vi "Copy To IMAQ.vi"() -> ()   [LabVIEW 2020]
uses:
  LabVIEW/g_ar_toolkit.image/Raw Memory Information.ctl
  LabVIEW/g_ar_toolkit.image/Raw Memory Information Dimension.ctl
  LabVIEW/g_ar_toolkit.image/DrawImageToPictureARGB.vi
  LabVIEW/g_ar_toolkit.image/NewImageARGB.vi/3321fa97-f432-4e1e-8db9-a0df79aed21b.vi
  LabVIEW/g_ar_toolkit.image/ARGB Colour to U32 Pixel Value.vi
  LabVIEW/g_ar_toolkit.image/DrawImageToPictureARGB.vi/8cd07b1b-062e-4fe4-9e87-2eb3dc89fe0e.vi
  LabVIEW/g_ar_toolkit.image/CopyImageToRawMemoryARGB.vi/01eda17f-9221-4e43-bf47-cf9d986167a3.vi
  LabVIEW/g_ar_toolkit.common/Module Path.vi
  <vilib>/Utility/error.llb/Error Cluster From Error Code.vi
  <vilib>/vision/EDVR.llb/IMAQ ImageToEDVR 2D U32.vi
  LabVIEW/g_ar_toolkit.image/g_ar_toolkit.image.lvlib
  LabVIEW/g_ar_toolkit.image/NewImageARGBArray.vi
panel:
  in  "Mode":T1(ring)
  out "IMAQ":T2(plugin-control)
  out "Input":picture
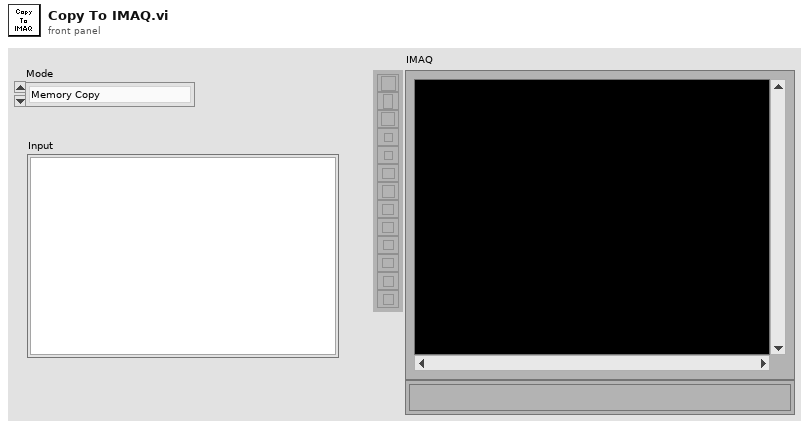
[diagram p1: front panel]
types:
  T1 = enum16{"Memory Copy", "EDVR Access", "Array Values"}
  T2 = typedef "IMAQ Image.ctl" = refnum<image>
  T3 = typedef "Image Type" = u32
  T4 = typedef "g_ar_toolkit.image.lvlib/ARGB Image.ctl" = refnum<data-value>
  T5 = enum32{"Map Pixel Pointer", "Unmap Pixel Pointer", "Get Pixels Infos"}
  T6 = typedef "g_ar_toolkit.image.lvlib/Raw Memory Information.ctl" = cluster{"Memory Address":u64, "Dimension 0":T7, "Dimension 1":T7}
  T7 = typedef "g_ar_toolkit.image.lvlib/Raw Memory Information Dimension.ctl" = cluster{"Size":u16, "Stride":u32}
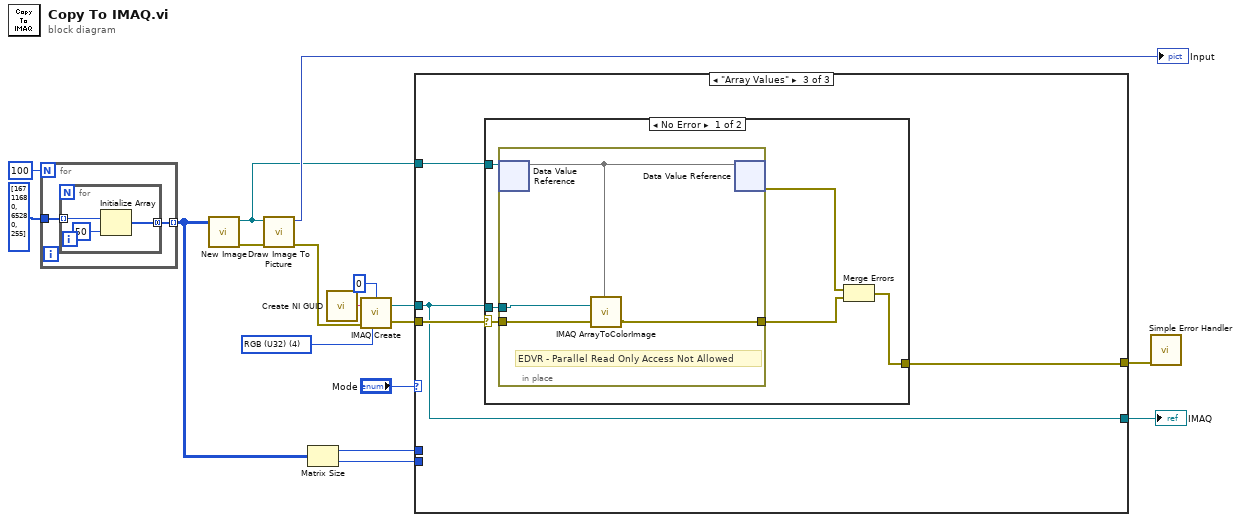
[diagram p0: block diagram]
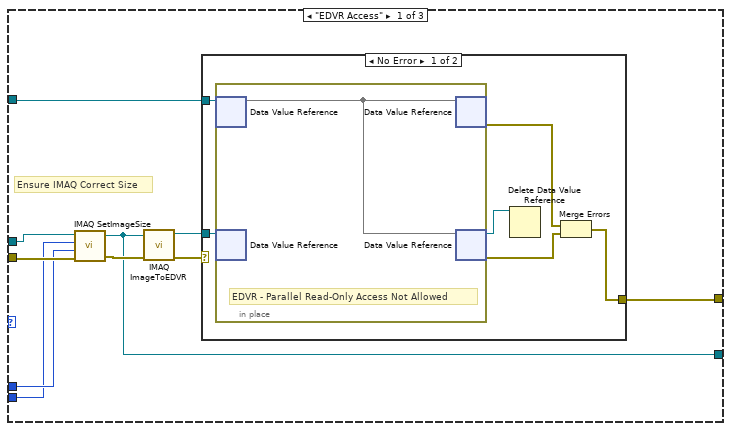
[diagram p2: hidden frame]
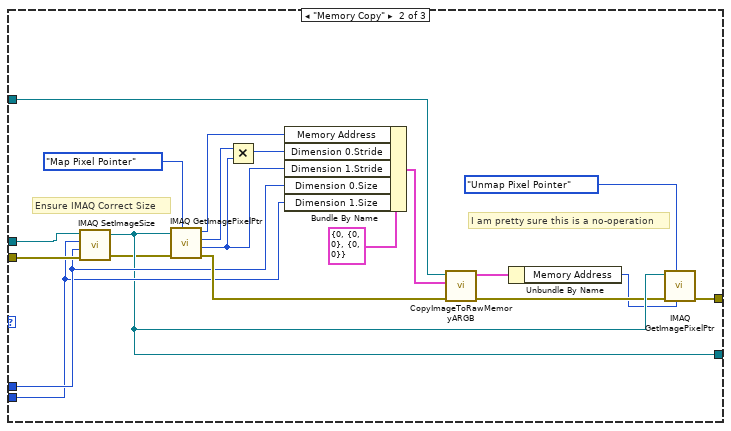
[diagram p4: hidden frame]
diagram:
  w15 = T3 4 items=["Grayscale (U8)", "Grayscale (I16)", "Grayscale (SGL)", "Complex (CSG)", "RGB (U32)", "HSL (U32)", "RGB (U64)", "Grayscale (U16)"] ("Image Type")
  n1 = for {
    N: 100 -> [_]
    tunnel: u32[] [16711680, 65280, 255] ("color(black)") -> [w19]
    tunnel: [w18] -> w1 mode=indexing
    n2 = for {
      tunnel: w19 -> [w22] mode=indexing
      tunnel: [w20] -> w18 mode=concatenating
      n3 = Initialize Array(w22, 50 ("dimension size")) -> (w20:u32[])
    }
  }
  n4 = call-poly "New Image.vi"("U32 ARBG Data  (Default: Empty)"=w1) -> ("error out"=w3:errorcluster, "New ARGB Image"=w2:T4)  [unwired: 9 in]
  n5 = call-poly "Draw Image To Picture.vi"("error in (no error)"=w3, "ARGB Image Source"=w2) -> ("error out"=w9:errorcluster, "Picture"=→"Input":picture)  [unwired: 8 in]
  n6 = Matrix Size(0:w1) -> (1:w11:i32, 2:w10:i32)
  n7 = call <vilib>:"Create NI GUID.vi"() -> ("NI GUID"=w5:string)
  n8 = call "IMAQ Create"("Border Size"=0, "Image Name"=w5, "Image Type"=w15, "error in (no error)"=w9) -> ("New Image"=w12:T2, "error out"=w13:errorcluster)  [unwired: 1 in]
  n9 = case shown="\"Array Values\"" "Mode" {
    tunnel: w13 -> [w29 w59 w64]
    tunnel: w12 -> [w28 w58 w61]
    tunnel: w11 -> [w24 w57 _]
    tunnel: w10 -> [w23 w56 _]
    tunnel: [w26 w55 w61] -> w7
    tunnel: [w27 w54 w62] -> w6
    tunnel: w2 -> [w25 w53 w63]
    frame "EDVR Access" {
      # "Ensure IMAQ Correct Size"
      n10 = call "IMAQ SetImageSize"("error in (no error)"=w29, "Y Resolution"=w24, "X Resolution"=w23, "Image"=w28) -> ("error out"=w32:errorcluster, "Image Out"=w26:T2)  [unwired: 1 in]
      n11 = call-poly <vilib>:"IMAQ ImageToEDVR.vi"("error out"=w32, "Image"=w26) -> ("error out"=w30:errorcluster, "EDVR 2D U32"=w31:refnum<data-value>)  [unwired: 7 in, 1 out]
      n12 = case shown="No Error" w30 {
        selector: w30 -> [_ w40]
        tunnel: w31 -> [w38 _]
        tunnel: [w34 w40] -> w27
        tunnel: w25 -> [w33 _]
        frame No Error {
          n13 = in-place {
            # "EDVR - Parallel Read-Only Access Not Allowed"
            n14 = in-place-dvr #1(w33) -> (w39:u32[][])  [unwired: 1 out]
            n15 = in-place-dvr #2(w38) -> ()  [unwired: 2 out]
            n16 = in-place-dvr #1(w39) -> (w36:errorcluster)  [unwired: 1 out]
            n17 = in-place-dvr #2(w39) -> (w37:refnum<data-value>, w35:errorcluster)
          }
          n18 = Delete Data Value Reference(data value reference=w37) -> ()  [unwired: 1 in, 2 out]
          n19 = Merge Errors(w36, w35) -> (w34:errorcluster)
        }
        frame Error {
        }
      }
    }
    frame "Memory Copy" {
      # "Ensure IMAQ Correct Size"
      # "I am pretty sure this is a no-operation"
      n20 = call "IMAQ SetImageSize"("error in (no error)"=w59, "Y Resolution"=w57, "X Resolution"=w56, "Image"=w58) -> ("error out"=w47:errorcluster, "Image Out"=w55:T2)  [unwired: 1 in]
      n21 = call "IMAQ GetImagePixelPtr"("Function"=T5."Map Pixel Pointer", "error in (no error)"=w47, "Image"=w55) -> ("error out"=w60:errorcluster, "Pixel Size (Bytes)"=w41:i32, "LineWidth(Pixels)"=w49:i32, "Pixel Pointer out"=w52:u64)  [unwired: 3 in, 2 out]
      n22 = Multiply(x=w49, y=w41) -> (x*y=w42:i32)
      n23 = Bundle By Name(cluster=T6 {"Memory Address"=0, "Dimension 0"={"Size"=0, "Stride"=0}, "Dimension 1"={"Size"=0, "Stride"=0}} ("Source"), "Memory Address"=w52, "Dimension 0.Stride"=w42, "Dimension 1.Stride"=w41, "Dimension 0.Size"=w57, "Dimension 1.Size"=w56) -> (w46:T6)
      n24 = call "CopyImageToRawMemoryARGB.vi"("error in (no error)"=w60, "Destination"=w46, "ARGB Image Source"=w53) -> ("error out"=w45:errorcluster, "Destination (Duplcate)"=w44:T6)  [unwired: 7 in]
      n25 = Unbundle By Name(w44) -> ("Memory Address"=w43:u64)
      n26 = call "IMAQ GetImagePixelPtr"("Pixel Pointer in"=w43, "Function"=T5."Unmap Pixel Pointer", "error in (no error)"=w45, "Image"=w55) -> ("error out"=w54:errorcluster)  [unwired: 2 in, 5 out]
    }
    frame "Array Values" {
      n27 = case shown="No Error" w64 {
        selector: w64 -> [w66 w75]
        tunnel: w63 -> [w70 _]
        tunnel: [w68 w75] -> w62
        tunnel: w61 -> [w67 _]
        frame No Error {
          n28 = in-place {
            in-place-border: w67 -> [w74]
            in-place-border: w66 -> [w73]
            in-place-border: [w71] -> w65
            # "EDVR - Parallel Read Only Access Not Allowed"
            n29 = in-place-dvr #3(w70) -> (w72:u32[][])  [unwired: 1 out]
            n30 = call "IMAQ ArrayToColorImage"("Image Pixels (U32)"=w72, "Image"=w74, "error in (no error)"=w73) -> ("error out"=w71:errorcluster)  [unwired: 2 in, 1 out]
            n31 = in-place-dvr #3(w72) -> (w69:errorcluster)  [unwired: 1 out]
          }
          n32 = Merge Errors(w69, w65) -> (w68:errorcluster)
        }
        frame Error {
        }
      }
    }
  }
  "IMAQ" <- w7
  n33 = call <vilib>:"Simple Error Handler.vi"("error in (no error)"=w6) -> ()  [unwired: 4 in, 5 out]
